vi "view.vi"() -> ()   [LabVIEW 2016]
uses:
  common_serial_tcpextended/common_serialprotocols/Configuration/SerialConfig.ctl
  common_serial_tcpextended/common_serialprotocols/Configuration/SerialProtocol.ctl
  common_serial_tcpextended/common_serialprotocols/Configuration/ProtocolParameters.ctl
  common_serial_tcpextended/common_serialprotocols/Configuration/SerialMessageParameters.ctl
  common_serial_tcpextended/common_ascii_tcp/tcpTypedefs/TCPSettings.ctl
  typedefs/WarningStatusFlag.ctl
  typedefs/AlarmStatusFlag.ctl
  typedefs/PumpStatusFlag.ctl
  typedefs/ControlStatusMode.ctl
  typedefs/ControlSensor.ctl
  CoolerController/typeOfWarning.ctl
  typedefs/ChillerStatus.ctl
  typedefs/ExternalSensorStatus.ctl
  CoolerController/CoolerControler.lvclass
  common_serial_tcpextended/CommunicatorClients/TCP/TCPCommunication.lvclass
  C:/Users/aanania/Documents/ss_atCooler/common_serial_tcpextended/Communicator/Communicator.lvclass
  common_serial_tcpextended/common_ascii_tcp/TCPClient/TCPClient.lvclass
  common_serial_tcpextended/common_ascii_tcp/TCPClient/TCPClient.lvclass/TCPClient.ctl
  common_serial_tcpextended/CommunicatorClients/TCP/TCPCommunication.lvclass/TCPCommunication.ctl
  common_serial_tcpextended/CommunicatorClients/Serial/SerialCommunication.lvclass
  common_serial_tcpextended/common_serialprotocols/SerialCommunicator/SerialCommunicator.lvclass
  common_serial_tcpextended/common_serialprotocols/SerialProtocolFactory/SerialProtocolFactory/SerialProtocolFactory.lvclass
  C:/Users/aanania/Documents/ss_atCooler/common_serial_tcpextended/common_serialprotocols/SerialProtocolFactory/ISerialProtocolFactory/ISerialProtocolFactory.lvclass
  common_serial_tcpextended/common_serialprotocols/SerialCommunicator/SerialCommunicator.lvclass/SerialCommunicator.ctl
  common_serial_tcpextended/CommunicatorClients/Serial/SerialCommunication.lvclass/SerialCommunication.ctl
  CoolerController/CoolerControler.lvclass/CoolerControler.ctl
  typedefs/readTempreature.ctl
  typedefs/typeOfError.ctl
  common_serial_tcpextended/common_serialprotocols/SerialProtocols.lvlib
  common_serial_tcpextended/common_ascii_tcp/tcp.lvlib
panel:
  in  "Communication Protocol":enum32{"TCP", "Serial"}(radio)
  in  "Configuration":enum32{"TCP", "Serial"}(tab)
  in  "tcpSettings":T1={"IP"="127.0.0.1", "port"=50000, "connection_timeout "=1500, "reading_timeout"=1500, "writing_timeout"=1500}
  in  "SerialConfig":T2={"Serial Protocol"=enum."RS232", "Protocol Parameters"={"VISA resource name"="ASRL11::INSTR", "Baud Rate"=9600, "Data Bits"=8, "Parity"=enum."None", "Flow Control"=1, "Stop Bits"=10, "Timeout (ms)"=1000}, "Serial Message Parameters"={"Byte Count"=200, "Enable Termination Character"=FALSE, "Termination Char"=13}} {"Serial Message Parameters"."Termination Char" format="%x"; "Protocol Parameters"."Stop Bits" items=["1.0"=10, "1.5"=15, "2.0"=20]; "Protocol Parameters"."Flow Control" items=["None", "XON/XOFF", "RTS/CTS", "XON/XOFF & RTS/CTS", "DTR/DSR", "XON/XOFF & DTR/DSR"]; "Protocol Parameters"."Data Bits" min=5 max=8 step=1}
  out "CS":T6
  out "AS":T7
  out "WS":T8
  out "PS":T9
  out "errors2":string
  out "errors3":string
  out "warnings":string
  out "AlarmStatus":string
  out "flow":sgl
  out "ambientTemperature":sgl
  out "supplyTemperature":sgl
  out "Temperature":sgl
  out "ControlSensor":T10
  out "Up time":u32
  out "Fan Speed 1":sgl
  out "Fan Speed 2":sgl
  out "Fan Speed 3":sgl
  out "Fan Speed 4":sgl
  in  "readFanSpeed":bool
  in  "readWarningStatus":bool
  in  "readAlarmStatus 3":bool
  in  "readAlarmStatus 2":bool
  in  "readAlarmStatus":bool
  in  "readProcessFlow":bool
  in  "readAmbientTemperature":bool
  in  "readSupplyTemperature":bool
  in  "readSetTemperature":bool
  in  "readControlSensor":bool
  in  "readSerialWatchDog":bool
  in  "readUnitUpTime":bool
  out "Connected":bool
  in  "stop":bool
  in  "disconnect":bool
  in  "connect":bool
  in  "temperature in":sgl
  in  "ControlSensor 2":T10
  in  "External Sensor Status":T11
  out "OKExternSensor":bool
  out "OKControlSensor":bool
  out "OKTemperature":bool
  out "OKWarning":bool
  out "OKChillerStatus":bool
  in  "ChillerStatus in":T12
  in  "setExternSensor":bool
  in  "setControlSensor":bool
  in  "setControlTemperature":bool
  in  "setChillerStatus":bool
  in  "Low":sgl
  in  "High":sgl
  in  "typeOfWarning":T13
  in  "setWarningOrAlarm":bool
  out "error out":errorcluster
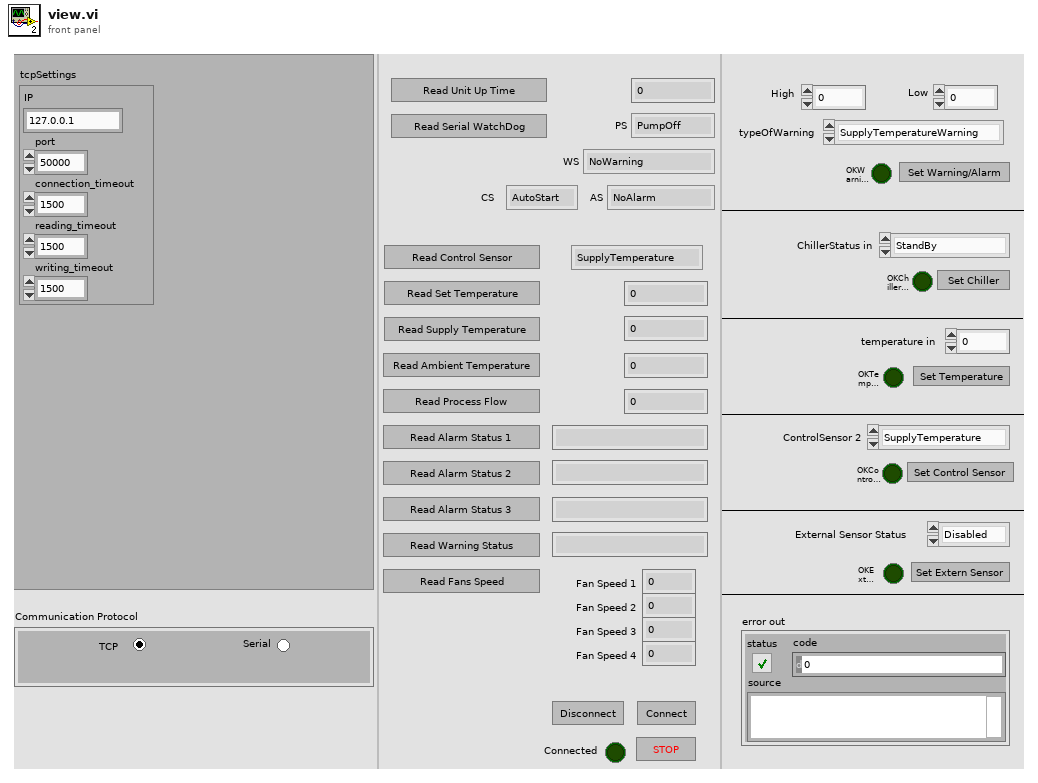
[diagram p1: front panel]
types:
  T1 = typedef "tcp.lvlib/TCPSettings.ctl" = cluster{"IP":string, "port":u16, "connection_timeout ":i32, "reading_timeout":i32, "writing_timeout":i32}
  T2 = typedef "SerialProtocols.lvlib/SerialConfig.ctl" = cluster{"Serial Protocol":T3, "Protocol Parameters":T4, "Serial Message Parameters":T5}
  T3 = typedef "SerialProtocols.lvlib/SerialProtocol.ctl" = enum16{"RS232", "RS485", "SerialSimulator"}
  T4 = typedef "SerialProtocols.lvlib/ProtocolParameters.ctl" = cluster{"VISA resource name":refnum<visa-resource-name>, "Baud Rate":u32, "Data Bits":u16, "Parity":enum16{"None", "Odd", "Even", "Mark", "Space"}, "Flow Control":u16, "Stop Bits":u16, "Timeout (ms)":u32}
  T5 = typedef "SerialProtocols.lvlib/SerialMessageParameters.ctl" = cluster{"Byte Count":u32, "Enable Termination Character":bool, "Termination Char":u8}
  T6 = typedef "ControlStatusMode.ctl" = enum16{"AutoStart", "Standby", "Run", "Safety", "Test"}
  T7 = typedef "AlarmStatusFlag.ctl" = enum16{"NoAlarm", "AlarmPresent"}
  T8 = typedef "WarningStatusFlag.ctl" = enum16{"NoWarning", "WarningPresent"}
  T9 = typedef "PumpStatusFlag.ctl" = enum16{"PumpOff", "PumpOn"}
  T10 = typedef "ControlSensor.ctl" = enum16{"SupplyTemperature", "ReturnTemperature", "ExtRTD", "ExternalTermistor"}
  T11 = typedef "ExternalSensorStatus.ctl" = enum16{"Disabled", "Enabled"}
  T12 = typedef "ChillerStatus.ctl" = enum16{"StandBy", "Run"}
  T13 = typedef "typeOfWarning.ctl" = enum16{"SupplyTemperatureWarning", "AmbientTemperatureWarning", "lowFlowWarning", "SupplyTemperatureAlarm", "AmbientTemperatureAlarm", "lowFlowAlarm"}
  T14 = typedef "readTempreature.ctl" = enum16{"SetTemperature", "AmbientTemperature", "SupplyTemperature", "ExternalRTDTemperature", "ReturnTemperature", "ExternalThermistor"}
  T15 = typedef "typeOfError.ctl" = enum16{"AlarmStateLevel1", "AlarmStateLevel21", "AlarmStateLevel22", "WarningStateLevel1"}
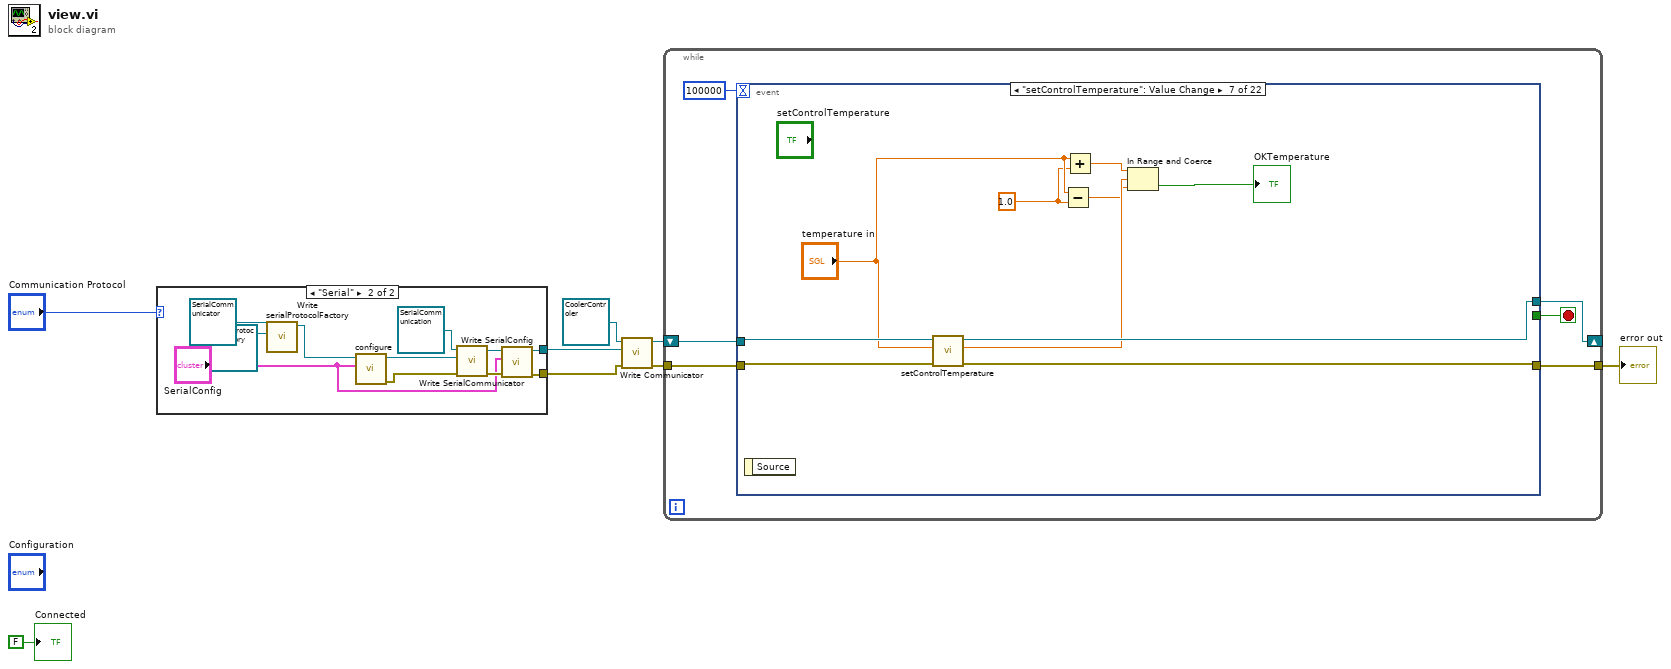
[diagram p0: block diagram]
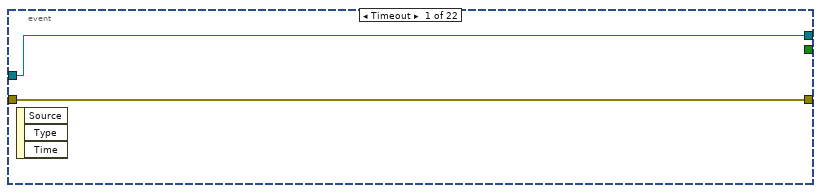
[diagram p2: hidden frame]
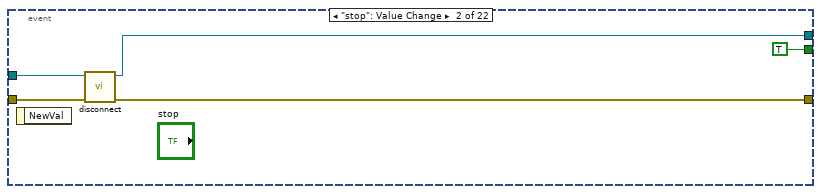
[diagram p3: hidden frame]
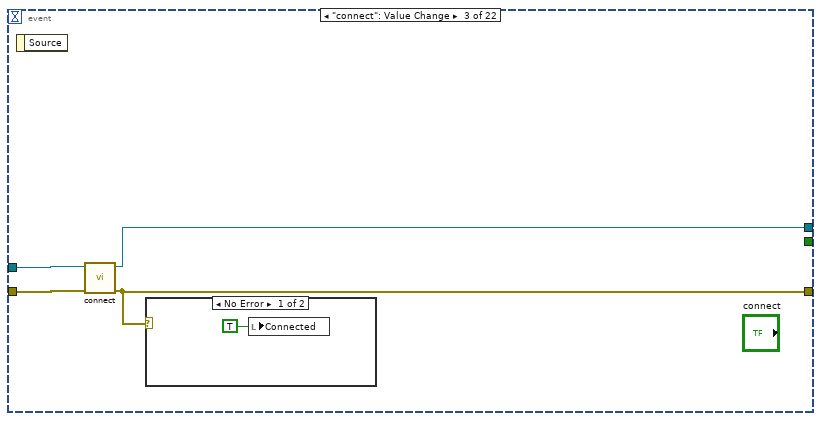
[diagram p4: hidden frame]
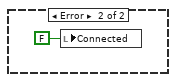
[diagram p5: hidden frame]
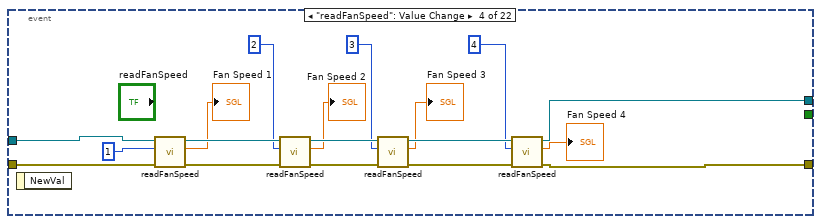
[diagram p6: hidden frame]
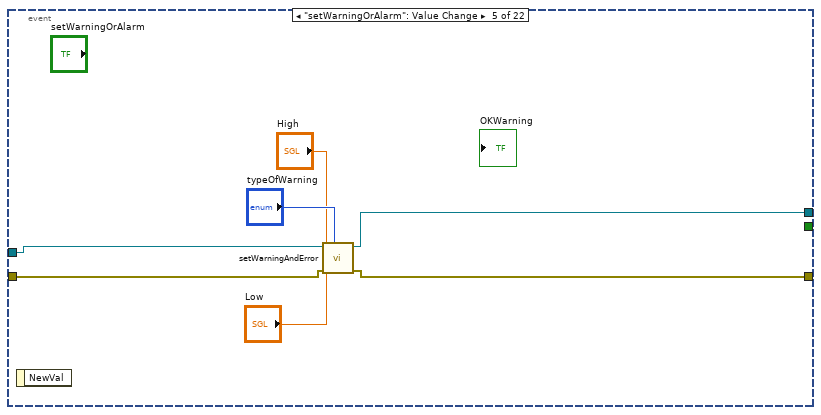
[diagram p7: hidden frame]
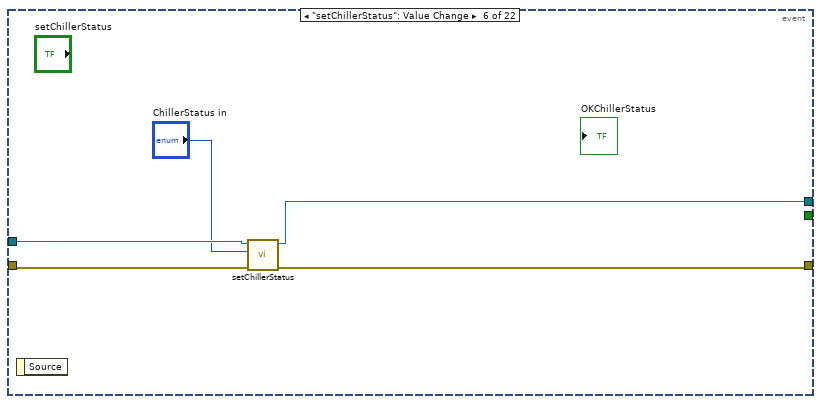
[diagram p8: hidden frame]
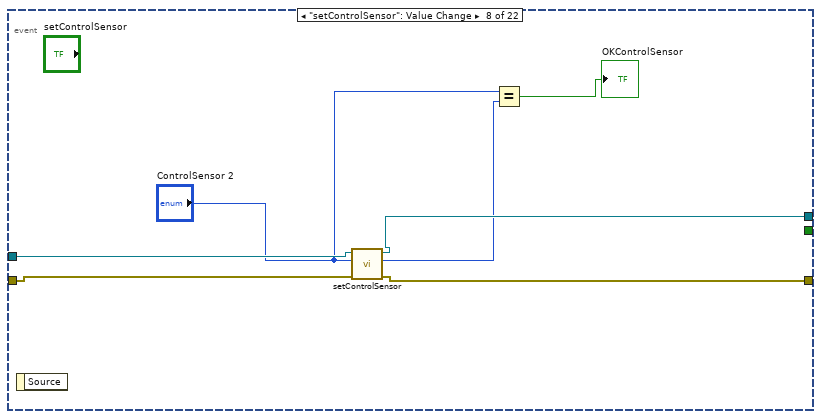
[diagram p9: hidden frame]
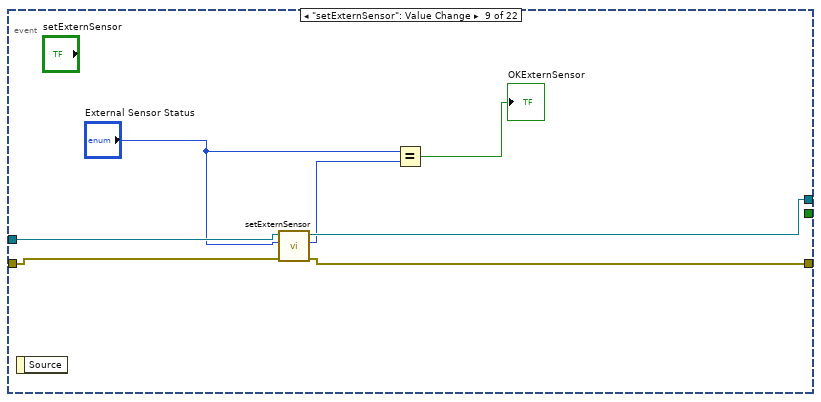
[diagram p10: hidden frame]
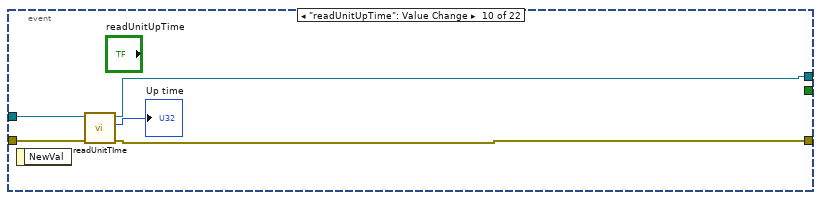
[diagram p11: hidden frame]
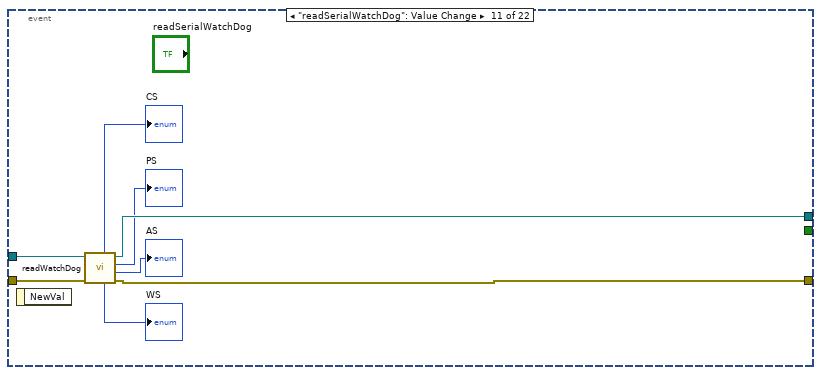
[diagram p12: hidden frame]
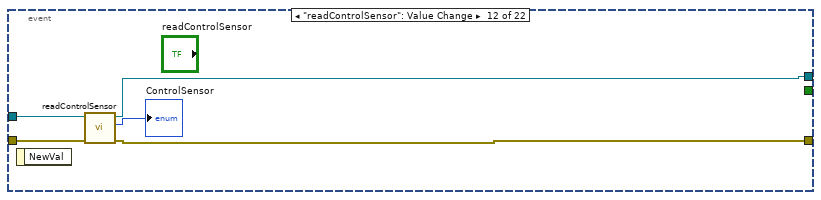
[diagram p13: hidden frame]
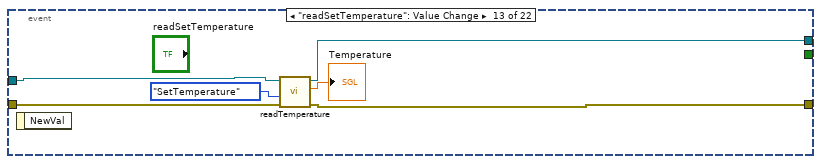
[diagram p14: hidden frame]
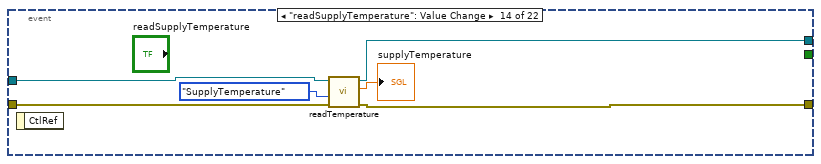
[diagram p15: hidden frame]
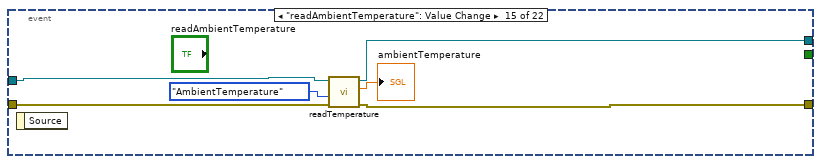
[diagram p16: hidden frame]
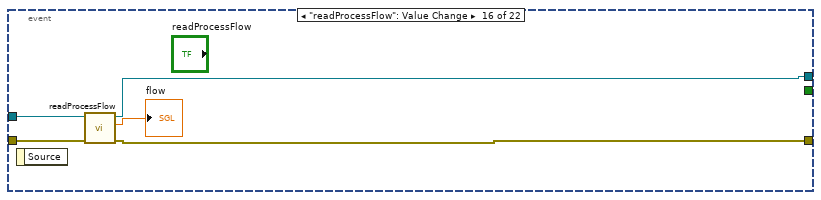
[diagram p17: hidden frame]
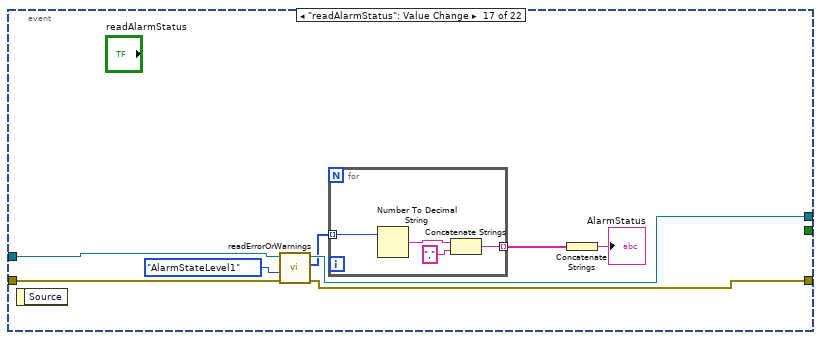
[diagram p18: hidden frame]
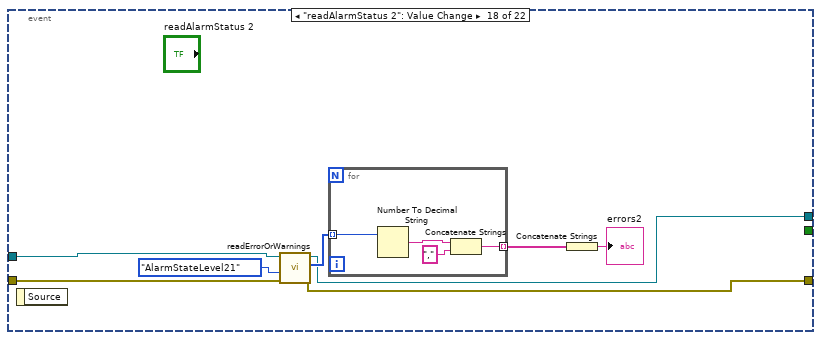
[diagram p19: hidden frame]
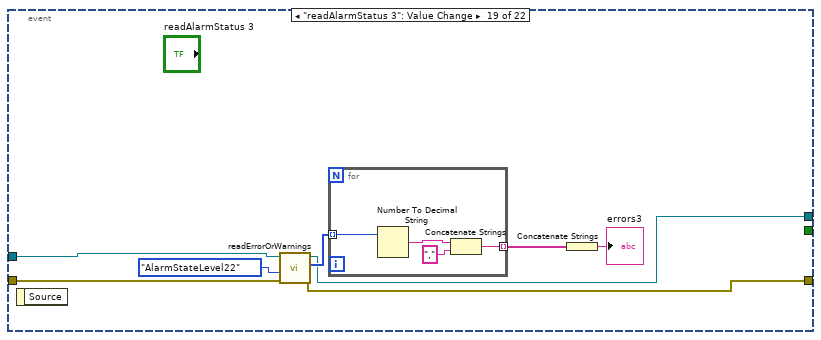
[diagram p20: hidden frame]
diagram:
  n1 = case shown="\"Serial\"" "Communication Protocol" {
    tunnel: [w11 w17] -> w4
    tunnel: [w9 w18] -> w1
    frame "TCP", Default {
      n2 = call "Write tcpSettings.vi"("tcpSettings"="tcpSettings", "TCPClient in"=refnum<class "TCPClient.lvclass"> refnum ("tcp.lvlib:TCPClient.lvclass")) -> ("error out"=w10:errorcluster, "TCPClient out"=w12:refnum<class "TCPClient.lvclass">)  [unwired: 8 in]
      n3 = call "Write TCPClient.vi"("error in (no error)"=w10, "tcp.lvlib:TCPClient.lvclass"=w12, "TCPClient in"=refnum<class "TCPCommunication.lvclass"> refnum ("TCPCommunication.lvclass")) -> ("error out"=w9:errorcluster, "TCPClient out"=w11:refnum<class "TCPCommunication.lvclass">)  [unwired: 7 in]
    }
    frame "Serial" {
      n4 = call "Write serialProtocolFactory.vi"("serialProtocolFactory"=refnum<class "SerialProtocolFactory.lvclass"> refnum ("SerialProtocols.lvlib:SerialProtocolFactory.lvclass"), "SerialCommunicator in"=refnum<class "SerialCommunicator.lvclass"> refnum ("SerialProtocols.lvlib:SerialCommunicator.lvclass")) -> ("SerialCommunicator out"=w22:refnum<class "SerialCommunicator.lvclass">)  [unwired: 9 in]
      n5 = call-dynamic "configure.vi"("SerialConfig"="SerialConfig", "SerialCommunicator in"=w22) -> ("error out"=w24:errorcluster, "SerialCommunicator out"=w25:refnum<class "SerialCommunicator.lvclass">)  [unwired: 8 in]
      n6 = call "Write SerialCommunicator.vi"("error in (no error)"=w24, "SerialProtocols.lvlib:SerialCommunicator.lvclass"=w25, "SerialClient in"=refnum<class "SerialCommunication.lvclass"> refnum ("SerialCommunication.lvclass")) -> ("error out"=w19:errorcluster, "SerialClient out"=w20:refnum<class "SerialCommunication.lvclass">)  [unwired: 7 in]
      n7 = call "Write SerialConfig.vi"("error in (no error)"=w19, "Serial"="SerialConfig", "SerialCommunication in"=w20) -> ("error out"=w18:errorcluster, "SerialCommunication out"=w17:refnum<class "SerialCommunication.lvclass">)  [unwired: 7 in]
    }
  }
  n8 = call "Write Communicator.vi"("error in (no error)"=w1, "Communicator.lvclass"=w4, "CoolerControler in"=refnum<class "CoolerControler.lvclass"> refnum) -> ("error out"=w2:errorcluster, "CoolerControler out"=w3:refnum<class "CoolerControler.lvclass">)  [unwired: 7 in]
  n9 = while {
    shift-right: [w27] -> _
    shift-left: w3 -> [w30]
    tunnel: w2 -> [w29]
    tunnel: [w28] -> w7
    stop <- w32 stop-if-true
    n10 = event shown="[6] \"setControlTemperature\": Value Change" {
      selector: _ -> [_ _ _ _ _ _ _ _ _ _ _ _ _ _ _ _ _ _ _ _ _ _]
      dyn-events: _ -> [_ _ _ _ _ _ _ _ _ _ _ _ _ _ _ _ _ _ _ _ _ _]
      timeout: 100000 -> [_ _ _ _ _ _ _ _ _ _ _ _ _ _ _ _ _ _ _ _ _ _]
      tunnel: [_ TRUE _ _ _ _ _ _ _ _ _ _ _ _ _ _ _ _ _ _ _ _] -> w32
      tunnel: w30 -> [w34 w38 w43 w63 w69 w75 w85 w92 w99 w104 w111 w117 w123 w127 w134 w140 w147 w157 w169 w181 w192 w196]
      tunnel: w29 -> [w33 w35 w40 w62 w70 w74 w84 w91 w98 w103 w112 w116 w122 w126 w133 w139 w148 w156 w168 w180 w189 w195]
      tunnel: [w33 w36 w41 w60 w67 w73 w83 w90 w97 w101 w109 w115 w121 w125 w132 w138 w145 w155 w167 w179 w193 w195] -> w28
      tunnel: [w34 w37 w42 w61 w68 w72 w82 w89 w96 w102 w110 w114 w120 w124 w131 w137 w144 w154 w166 w178 w191 w196] -> w27
      event Timeout {
        n11 = event-data() -> ()  [unwired: 1 in, 3 out]
      }
      event "stop": Value Change {
        n12 = event-data() -> ()  [unwired: 1 in, 1 out]
        n13 = call "disconnect.vi"("error in (no error)"=w35, "CoolerControler in"=w38) -> ("error out"=w36:errorcluster, "CoolerControler out"=w37:refnum<class "CoolerControler.lvclass">)  [unwired: 8 in]
      }
      event "connect": Value Change {
        n14 = event-data() -> ()  [unwired: 1 in, 1 out]
        n15 = call "connect.vi"("error in (no error)"=w40, "CoolerControler in"=w43) -> ("error out"=w41:errorcluster, "CoolerControler out"=w42:refnum<class "CoolerControler.lvclass">)  [unwired: 8 in]
        n16 = case shown="No Error" w41 {
          frame No Error {
            n17 = local write "Connected"(TRUE ("Connected")) -> ()
          }
          frame Error {
            n18 = local write "Connected"(FALSE ("Connected")) -> ()
          }
        }
      }
      event "readFanSpeed": Value Change {
        n19 = event-data() -> ()  [unwired: 1 in, 1 out]
        n20 = call "readFanSpeed.vi"("error in (no error)"=w62, "fanNumber"=1, "CoolerControler in"=w63) -> ("error out"=w57:errorcluster, "fanSpeed"=→"Fan Speed 1":sgl, "CoolerControler out"=w56:refnum<class "CoolerControler.lvclass">)  [unwired: 6 in]
        n21 = call "readFanSpeed.vi"("error in (no error)"=w57, "fanNumber"=2, "CoolerControler in"=w56) -> ("error out"=w58:errorcluster, "fanSpeed"=→"Fan Speed 2":sgl, "CoolerControler out"=w55:refnum<class "CoolerControler.lvclass">)  [unwired: 6 in]
        n22 = call "readFanSpeed.vi"("error in (no error)"=w58, "fanNumber"=3, "CoolerControler in"=w55) -> ("error out"=w59:errorcluster, "fanSpeed"=→"Fan Speed 3":sgl, "CoolerControler out"=w54:refnum<class "CoolerControler.lvclass">)  [unwired: 6 in]
        n23 = call "readFanSpeed.vi"("error in (no error)"=w59, "fanNumber"=4, "CoolerControler in"=w54) -> ("error out"=w60:errorcluster, "fanSpeed"=→"Fan Speed 4":sgl, "CoolerControler out"=w61:refnum<class "CoolerControler.lvclass">)  [unwired: 6 in]
      }
      event "setWarningOrAlarm": Value Change {
        n24 = event-data() -> ()  [unwired: 1 in, 1 out]
        n25 = call "setWarningAndError.vi"("typeOfWarning"="typeOfWarning", "error in (no error)"=w70, "Low"="Low", "High"="High", "CoolerControler in"=w69) -> ("error out"=w67:errorcluster, "CoolerControler out"=w68:refnum<class "CoolerControler.lvclass">)  [unwired: 3 in, 2 out]
      }
      event "setChillerStatus": Value Change {
        n26 = event-data() -> ()  [unwired: 1 in, 1 out]
        n27 = call "setChillerStatus.vi"("error in (no error)"=w74, "ChillerStatus in"="ChillerStatus in", "CoolerControler in"=w75) -> ("error out"=w73:errorcluster, "CoolerControler out"=w72:refnum<class "CoolerControler.lvclass">)  [unwired: 6 in, 1 out]
      }
      event "setControlTemperature": Value Change {
        w76 = sgl 1.0 ("y")
        n28 = event-data() -> ()  [unwired: 1 in, 1 out]
        n29 = call "setControlTemperature.vi"("error in (no error)"=w84, "temperature in"="temperature in", "CoolerControler in"=w85) -> ("error out"=w83:errorcluster, "temperature out"=w80:sgl, "CoolerControler out"=w82:refnum<class "CoolerControler.lvclass">)  [unwired: 6 in]
        n30 = Subtract(x="temperature in", y=w76) -> (x-y=w79:sgl)
        n31 = Add(x="temperature in", y=w76) -> (x+y=w78:sgl)
        n32 = In Range and Coerce(upper limit=w78, x=w80, lower limit=w79) -> (In Range?=→"OKTemperature":bool)  [unwired: 1 out]
      }
      event "setControlSensor": Value Change {
        n33 = event-data() -> ()  [unwired: 1 in, 1 out]
        n34 = call "setControlSensor.vi"("error in (no error)"=w91, "ControlSensor in"="ControlSensor 2", "CoolerControler in"=w92) -> ("error out"=w90:errorcluster, "ControlSensor out"=w86:T10, "CoolerControler out"=w89:refnum<class "CoolerControler.lvclass">)  [unwired: 6 in]
        n35 = Equal?(x="ControlSensor 2", y=w86) -> (x = y?=→"OKControlSensor":bool)
      }
      event "setExternSensor": Value Change {
        n36 = event-data() -> ()  [unwired: 1 in, 1 out]
        n37 = call "setExternSensor.vi"("error in (no error)"=w98, "ExternalSensorStatus"="External Sensor Status", "CoolerControler in"=w99) -> ("error out"=w97:errorcluster, "ExternalSensorStatus out"=w94:T11, "CoolerControler out"=w96:refnum<class "CoolerControler.lvclass">)  [unwired: 6 in]
        n38 = Equal?(x="External Sensor Status", y=w94) -> (x = y?=→"OKExternSensor":bool)
      }
      event "readUnitUpTime": Value Change {
        n39 = event-data() -> ()  [unwired: 1 in, 1 out]
        n40 = call "readUnitTIme.vi"("error in (no error)"=w103, "CoolerControler in"=w104) -> ("error out"=w101:errorcluster, "unitTime"=→"Up time":u32, "CoolerControler out"=w102:refnum<class "CoolerControler.lvclass">)  [unwired: 7 in]
      }
      event "readSerialWatchDog": Value Change {
        n41 = event-data() -> ()  [unwired: 1 in, 1 out]
        n42 = call "readWatchDog.vi"("error in (no error)"=w112, "CoolerControler in"=w111) -> ("error out"=w109:errorcluster, "AS"=→"AS":T7, "PS"=→"PS":T9, "CoolerControler out"=w110:refnum<class "CoolerControler.lvclass">, "WS"=→"WS":T8, "CS"=→"CS":T6)  [unwired: 4 in]
      }
      event "readControlSensor": Value Change {
        n43 = event-data() -> ()  [unwired: 1 in, 1 out]
        n44 = call "readControlSensor.vi"("error in (no error)"=w116, "CoolerControler in"=w117) -> ("error out"=w115:errorcluster, "ControlSensor"=→"ControlSensor":T10, "CoolerControler out"=w114:refnum<class "CoolerControler.lvclass">)  [unwired: 7 in]
      }
      event "readSetTemperature": Value Change {
        n45 = event-data() -> ()  [unwired: 1 in, 1 out]
        n46 = call "readTemperature.vi"("error in (no error)"=w122, "TemperatureType"=readTempreature."SetTemperature", "CoolerControler in"=w123) -> ("error out"=w121:errorcluster, "temperature"=→"Temperature":sgl, "CoolerControler out"=w120:refnum<class "CoolerControler.lvclass">)  [unwired: 6 in]
      }
      event "readSupplyTemperature": Value Change {
        n47 = event-data() -> ()  [unwired: 1 in, 1 out]
        n48 = call "readTemperature.vi"("error in (no error)"=w126, "TemperatureType"=readTempreature."SupplyTemperature", "CoolerControler in"=w127) -> ("error out"=w125:errorcluster, "temperature"=→"supplyTemperature":sgl, "CoolerControler out"=w124:refnum<class "CoolerControler.lvclass">)  [unwired: 6 in]
      }
      event "readAmbientTemperature": Value Change {
        n49 = event-data() -> ()  [unwired: 1 in, 1 out]
        n50 = call "readTemperature.vi"("error in (no error)"=w133, "TemperatureType"=readTempreature."AmbientTemperature", "CoolerControler in"=w134) -> ("error out"=w132:errorcluster, "temperature"=→"ambientTemperature":sgl, "CoolerControler out"=w131:refnum<class "CoolerControler.lvclass">)  [unwired: 6 in]
      }
      event "readProcessFlow": Value Change {
        n51 = event-data() -> ()  [unwired: 1 in, 1 out]
        n52 = call "readProcessFlow.vi"("error in (no error)"=w139, "CoolerControler in"=w140) -> ("error out"=w138:errorcluster, "flow"=→"flow":sgl, "CoolerControler out"=w137:refnum<class "CoolerControler.lvclass">)  [unwired: 7 in]
      }
      event "readAlarmStatus": Value Change {
        n53 = event-data() -> ()  [unwired: 1 in, 1 out]
        n54 = call "readErrorOrWarnings.vi"("error in (no error)"=w148, "typeOfError"=typeOfError."AlarmStateLevel1", "CoolerControler in"=w147) -> ("error out"=w145:errorcluster, "errorsArray"=w143:u16[], "CoolerControler out"=w144:refnum<class "CoolerControler.lvclass">)  [unwired: 6 in]
        n55 = for {
          tunnel: w143 -> [w150] mode=indexing
          tunnel: [w149] -> w142 mode=indexing
          n56 = Number To Decimal String(number=w150) -> (decimal integer string=w152:string)  [unwired: 1 in]
          n57 = Concatenate Strings(w152, "," ("string")) -> (w149:string)
        }
        n58 = Concatenate Strings(w142) -> (→"AlarmStatus":string)
      }
      event "readAlarmStatus 2": Value Change {
        n59 = event-data() -> ()  [unwired: 1 in, 1 out]
        n60 = call "readErrorOrWarnings.vi"("error in (no error)"=w156, "typeOfError"=typeOfError."AlarmStateLevel21", "CoolerControler in"=w157) -> ("error out"=w155:errorcluster, "errorsArray"=w159:u16[], "CoolerControler out"=w154:refnum<class "CoolerControler.lvclass">)  [unwired: 6 in]
        n61 = for {
          tunnel: w159 -> [w162] mode=indexing
          tunnel: [w161] -> w158 mode=indexing
          n62 = Number To Decimal String(number=w162) -> (decimal integer string=w164:string)  [unwired: 1 in]
          n63 = Concatenate Strings(w164, "," ("string")) -> (w161:string)
        }
        n64 = Concatenate Strings(w158) -> (→"errors2":string)
      }
      event "readAlarmStatus 3": Value Change {
        n65 = event-data() -> ()  [unwired: 1 in, 1 out]
        n66 = call "readErrorOrWarnings.vi"("error in (no error)"=w168, "typeOfError"=typeOfError."AlarmStateLevel22", "CoolerControler in"=w169) -> ("error out"=w167:errorcluster, "errorsArray"=w171:u16[], "CoolerControler out"=w166:refnum<class "CoolerControler.lvclass">)  [unwired: 6 in]
        n67 = for {
          tunnel: w171 -> [w174] mode=indexing
          tunnel: [w173] -> w170 mode=indexing
          n68 = Number To Decimal String(number=w174) -> (decimal integer string=w176:string)  [unwired: 1 in]
          n69 = Concatenate Strings(w176, "," ("string")) -> (w173:string)
        }
        n70 = Concatenate Strings(w170) -> (→"errors3":string)
      }
      event "readWarningStatus": Value Change {
        n71 = event-data() -> ()  [unwired: 1 in, 1 out]
        n72 = call "readErrorOrWarnings.vi"("error in (no error)"=w180, "typeOfError"=typeOfError."WarningStateLevel1", "CoolerControler in"=w181) -> ("error out"=w179:errorcluster, "errorsArray"=w183:u16[], "CoolerControler out"=w178:refnum<class "CoolerControler.lvclass">)  [unwired: 6 in]
        n73 = for {
          tunnel: w183 -> [w186] mode=indexing
          tunnel: [w185] -> w182 mode=indexing
          n74 = Number To Decimal String(number=w186) -> (decimal integer string=w188:string)  [unwired: 1 in]
          n75 = Concatenate Strings(w188, "," ("string")) -> (w185:string)
        }
        n76 = Concatenate Strings(w182) -> (→"warnings":string)
      }
      event "disconnect": Value Change {
        # "Clear in case it couldn't disconnect because it was disconnected"
        n77 = event-data() -> ()  [unwired: 1 in, 1 out]
        n78 = call "disconnect.vi"("error in (no error)"=w189, "CoolerControler in"=w192) -> ("error out"=w190:errorcluster, "CoolerControler out"=w191:refnum<class "CoolerControler.lvclass">)  [unwired: 8 in]
        n79 = local write "Connected"(FALSE ("Connected")) -> ()
        n80 = call <vilib>:"Clear Errors.vi"("error in (no error)"=w190) -> ("error out"=w193:errorcluster)  [unwired: 5 in, 1 out]
      }
      event "Communication Protocol": Value Change {
        n81 = event-data() -> ("NewVal"=w197:enum32{"TCP", "Serial"})  [unwired: 1 in]
        n82 = property on="Configuration" class="TabCtl (strict)"("Value"=w197) -> ()  [unwired: 2 in, 2 out]
      }
    }
  }
  "error out" <- w7
  "Connected" <- FALSE ("Connected")
